vi "recordStartPauseTime.vi"(8 "error in (no error)":errorcluster, 11 "Model in":refnum<class "Model.lvclass">) -> (0 "error out":errorcluster, 3 "Model out":refnum<class "Model.lvclass">)   [LabVIEW 2013, in "Model.lvclass"]
uses:
  Model.lvclass
  Model.lvclass/Model.ctl
  ApplicationElements/TestMonitor/TestMonitor.lvclass/TestMonitor.ctl
  ApplicationElements/TestMonitor/TestMonitor.lvclass
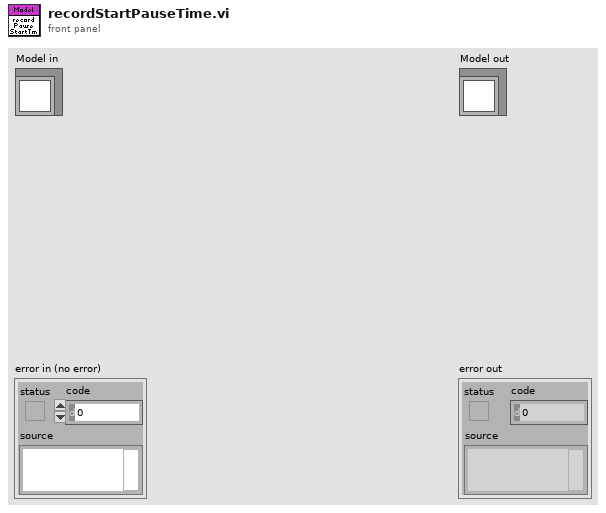
[diagram p1: front panel]
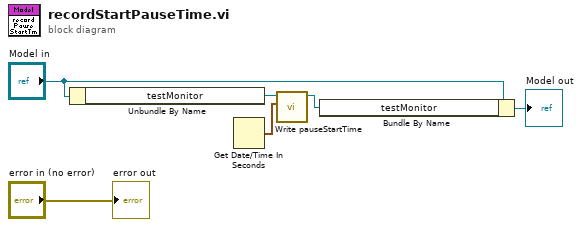
[diagram p0: block diagram]
diagram:
  n1 = Unbundle By Name("Model in") -> ("testMonitor"=w3:refnum<class "TestMonitor.lvclass">)
  n2 = Get Date/Time In Seconds() -> (seconds since 1Jan1904=w1:timestamp)
  n3 = call "Write pauseStartTime.vi"("pauseStartTime"=w1, "TestMonitor in"=w3) -> ("TestMonitor out"=w2:refnum<class "TestMonitor.lvclass">)  [unwired: 9 in]
  n4 = Bundle By Name(cluster="Model in", "testMonitor"=w2) -> (→"Model out":refnum<class "Model.lvclass">)
  "error out" <- "error in (no error)"
